vi "Open First Controller.vi"(7 "Enable Events (T)":bool=TRUE, 8 "Error In":errorcluster) -> (0 "Error Out":errorcluster, 2 "Event Registration Refnum":refnum<event-registration>, 3 "PS4 Controller Ref":T1)   [LabVIEW 2011, in "LMH-PS4.lvlib"]
doc: "Attempt to auto detect the PS4 controller by name (\"Wireless Controller\") and open a connection if it is found."
uses:
  LMH-PS4.lvlib
  Private/Type Defs/PS4 Controller Ref.ctl
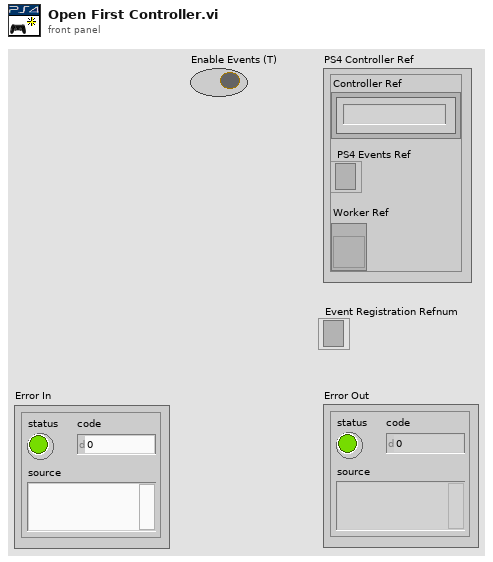
[diagram p1: front panel]
types:
  T1 = typedef "LMH-PS4.lvlib/PS4 Controller Ref.ctl" = cluster{"Controller Ref":refnum<k1>, "PS4 Events Ref":refnum<event-registration>, "Worker Ref":refnum<vi>}
  T2 = cluster{"axes total":u32, "buttons total":u32, "pov total":u32, "device name":string}[]
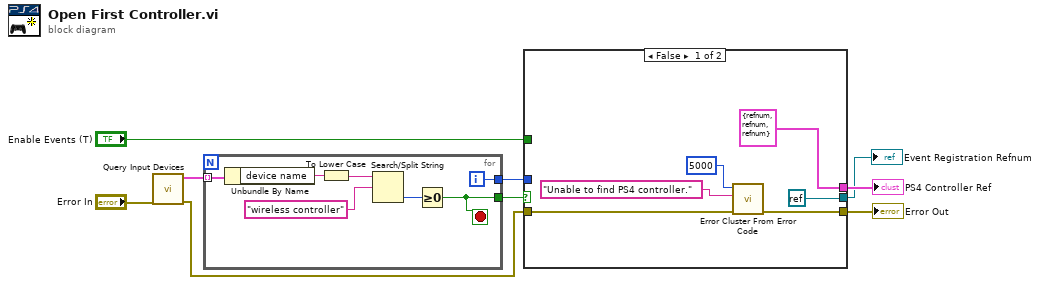
[diagram p0: block diagram]
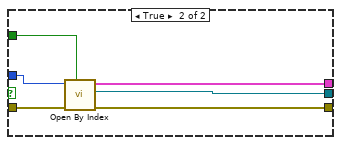
[diagram p2: hidden frame]
diagram:
  n1 = call <vilib>:"Query Input Devices.vi"("error in (no error)"="Error In") -> ("error out"=w6:errorcluster, "joystick info"=w9:T2)  [unwired: 7 in, 2 out]
  n2 = for {
    tunnel: w9 -> [w16] mode=indexing
    tunnel: [w11] -> w8
    tunnel: [w10] -> w7
    i -> [w10]
    stop <- w11 stop-if-true
    n3 = Unbundle By Name(w16) -> ("device name"=w13:string)
    n4 = To Lower Case(string=w13) -> (all lower case string=w12:string)
    n5 = Search/Split String(string=w12, search string/char (-)="wireless controller") -> (offset of match=w15:i32)  [unwired: 1 in, 2 out]
    n6 = Greater Or Equal To 0?(x=w15) -> (x >= 0?=w11:bool)
  }
  n7 = case shown="False" w8 {
    tunnel: w7 -> [_ w27]
    tunnel: w6 -> [w22 w28]
    tunnel: "Enable Events (T)" -> [_ w26]
    tunnel: [T1 {"Controller Ref"=refnum, "PS4 Events Ref"=refnum, "Worker Ref"=refnum} ("PS4 Controller Ref") w25] -> w4
    tunnel: [refnum<k0> refnum w24] -> w3
    tunnel: [w21 w23] -> w2
    frame False {
      n8 = call <vilib>:"Error Cluster From Error Code.vi"("error in (no error)"=w22, "error message (\"\")"="Unable to find PS4 controller.", "error code (0)"=5000) -> ("error out"=w21:errorcluster)  [unwired: 6 in]
    }
    frame True {
      n9 = call "Open By Index.vi"("Enable Events (T)"=w26, "Error In"=w28, "Device Index"=w27) -> ("Error Out"=w23:errorcluster, "PS4 Event Refs"=w24:refnum<event-registration>, "PS4 Controller Ref"=w25:T1)  [unwired: 6 in]
    }
  }
  "PS4 Controller Ref" <- w4
  "Event Registration Refnum" <- w3
  "Error Out" <- w2
